vi "queue_state_&_argument.vi"   [LabVIEW 2015]
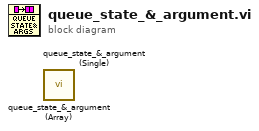
[diagram p0: block diagram]
diagram:
  n1 = call "queue_state_&_argument (Array).vi"() -> ()  [unwired: 10 in, 2 out]
  n2 = call "queue_state_&_argument (Single).vi"() -> ()  [unwired: 10 in, 2 out]
